vi "DAC Save Results.vi"(8 "error in":errorcluster, 9 "Log Details?":bool, 10 "tdms file":refnum<k34>, 11 "DAC Keller BNC in":refnum<class "DAC Keller BNC.lvclass">) -> (0 "error out":errorcluster)   [LabVIEW 2019, in "DAC.lvlib" / "DAC Keller BNC.lvclass"]
uses:
  DAC Keller BNC.lvclass
  C:/Users/krio/Documents/LV_Projects/test-stand/App/DAC/DAC.lvclass
  DAC.lvclass/DAC.ctl
  DAC Keller BNC.lvclass/DAC Keller BNC.ctl
  DAC.lvclass
  <vilib>/Analysis/NI_AALBase.lvlib
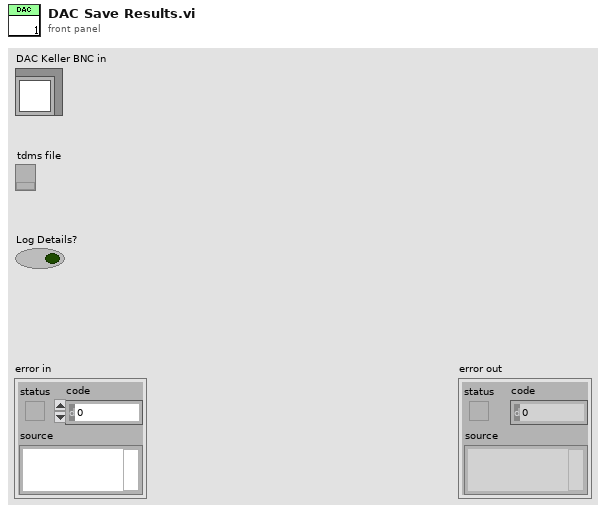
[diagram p1: front panel]
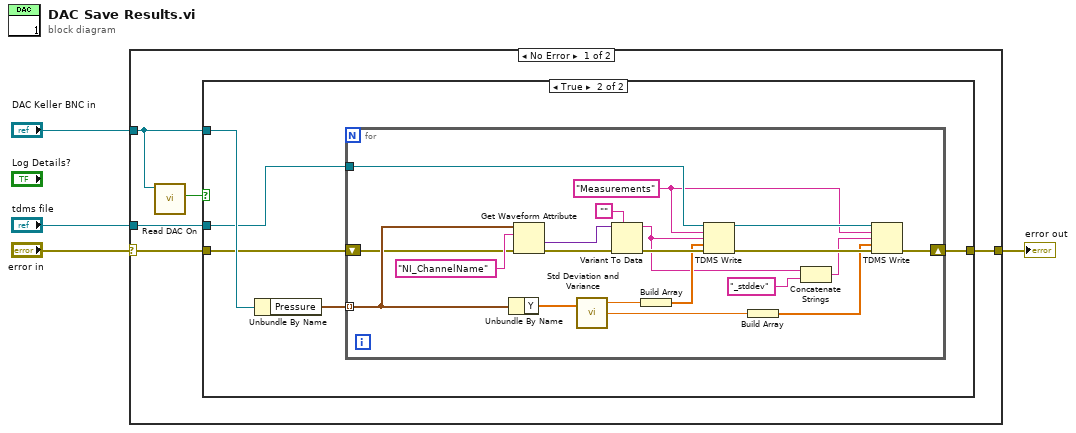
[diagram p0: block diagram]
diagram:
  n1 = case shown="No Error" "error in" {
    selector: "error in" -> [w6 w35]
    tunnel: "DAC Keller BNC in" -> [w9 _]
    tunnel: "tdms file" -> [w7 _]
    tunnel: [w5 w35] -> w1
    frame No Error {
      n2 = call "Read DAC On.vi"("DAC in"=w9) -> ("DAC On"=w8:bool)  [unwired: 8 in, 2 out]
      n3 = case shown="True" w8 {
        tunnel: w9 -> [_ w15]
        tunnel: w7 -> [_ w14]
        tunnel: w6 -> [w10 w12]
        tunnel: [w10 w11] -> w5
        frame False {
        }
        frame True {
          n4 = Unbundle By Name(w15) -> ("Pressure"=w13:waveform(dbl)[])
          n5 = for {
            tunnel: w14 -> [w34]
            tunnel: w13 -> [w30] mode=indexing
            shift-right: [w26] -> w11
            shift-left: w12 -> [w29]
            w16 = "Measurements" ("group name in (Untitled)")
            n6 = Unbundle By Name(w30) -> ("Y"=w25:dbl[])
            n7 = Get Waveform Attribute(4:w29, 6:"NI_ChannelName" ("name"), 7:w30) -> (0:w28:errorcluster, 1:w32:variant)  [unwired: 1 in, 2 out]
            n8 = call <vilib>:"Std Deviation and Variance.vi"("X"=w25) -> ("mean"=w24:dbl, "standard deviation"=w22:dbl)  [unwired: 1 in, 1 out]
            n9 = Variant To Data(error in=w28, type="", Variant=w32) -> (data=w19:string, error out=w27:errorcluster)
            n10 = Build Array(w24) -> (w23:dbl[])
            n11 = TDMS Write(0:w34, 5:w16, 7:w19, 9:w23, 11:w27) -> (4:w17:refnum<k34>, 15:w26:errorcluster)  [unwired: 1 in, 2 out]
            n12 = Build Array(w22) -> (w21:dbl[])
            n13 = Concatenate Strings(w19, "_stddev" ("string")) -> (w18:string)
            n14 = TDMS Write(0:w17, 5:w16, 7:w18, 9:w21) -> ()  [unwired: 2 in, 4 out]
          }
        }
      }
    }
    frame Error {
    }
  }
  "error out" <- w1
